vi "Yokogawa GX20 Acquire Continuous Measurement Data Example Ether Multiple.vi"() -> ()   [LabVIEW 2020]
doc: "This example shows how to configure multiple channels and acquire measurement data from multiple channels."
uses:
  <instrlib>/Yokogawa GX Series/Public/Data/Read Measurement Data (Analog NChan).vi
  <instrlib>/Yokogawa GX Series/Yokogawa GX Series.lvlib
panel:
  out "Chart":dbl[][](graph)
  in  "Parameters":T1(array[cluster])
  in  "Interval (1000)":u32=1000 min=25
  in  "Stop":bool
  # "(c) 2013-2018 Yokogawa Electric Corporation.  ALL RIGHTS RESERVED."
  # "ms"
  # "To execute this example, do below.\n1) Attach AI module to GX/GP/GM.\n2) Do Reconfiguring the GX/GP/GM (See User's Manual 1.24.2)\n3) Run this VI with valid VISA resource name (ex: \"TCPIP::192.168.0.2::34434::SOCKET\")"
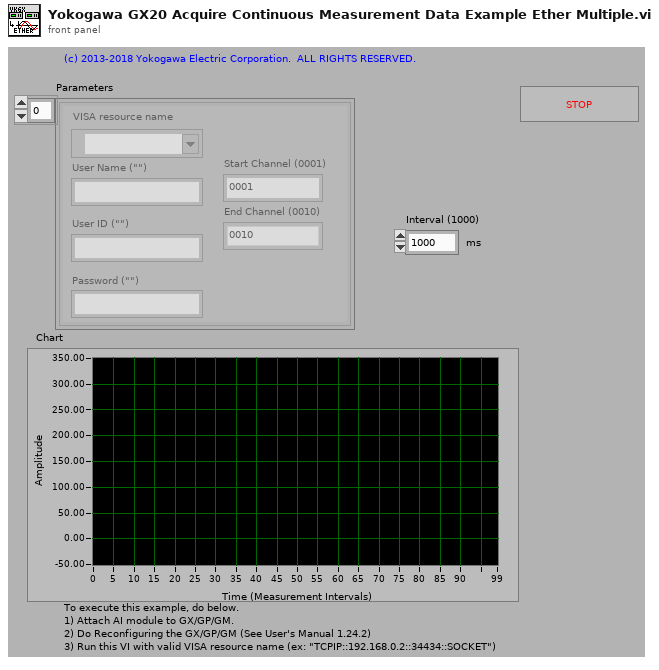
[diagram p1: front panel]
types:
  T1 = cluster{"VISA resource name":refnum<visa-resource-name>, "User Name (\"\")":string, "Password (\"\")":string, "Start Channel (0001) ":string, "End Channel (0010)":string, "User ID (\"\")":string}[]
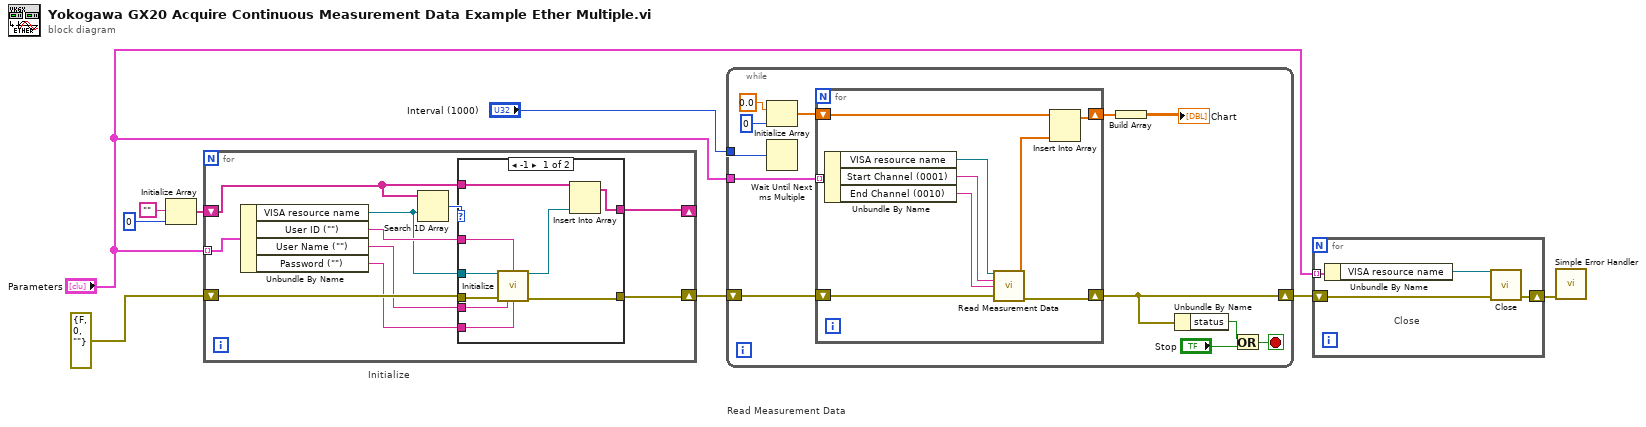
[diagram p0: block diagram]
diagram:
  # "Read Measurement Data"
  # "Initialize"
  n1 = Initialize Array("", 0) -> (w2:string[])
  n2 = for {
    tunnel: "Parameters" -> [w19] mode=indexing
    shift-right: [w17] -> w6
    shift-left: errorcluster {"status"=FALSE, "code"=0, "source"=""} ("error in (no error)") -> [w18]
    shift-right: [w14] -> _
    shift-left: w2 -> [w15]
    n3 = Unbundle By Name(w19) -> ("VISA resource name"=w10:refnum<visa-resource-name>, "User ID (\"\")"=w11:string, "User Name (\"\")"=w12:string, "Password (\"\")"=w13:string)
    n4 = Search 1D Array(1D array=w15, element=w10) -> (index of element=w16:i32)  [unwired: 1 in]
    n5 = case shown="-1" w16 {
      tunnel: w18 -> [w28 w29]
      tunnel: [w21 w29] -> w17
      tunnel: w12 -> [w27 _]
      tunnel: w13 -> [w26 _]
      tunnel: w10 -> [w25 _]
      tunnel: w15 -> [w24 w30]
      tunnel: [w23 w30] -> w14
      tunnel: w11 -> [w20 _]
      frame -1 {
        n6 = call <instrlib>:"Initialize.vi"("VISA resource name IN"=w25, "User ID (\"\")"=w20, "error in (no error)"=w28, "User Name (\"admin\")"=w27, "Password (\"\")"=w26) -> ("VISA resource name out"=w22:refnum<visa-resource-name>, "error out"=w21:errorcluster)  [unwired: 9 in]
        n7 = Insert Into Array(array=w24, new element=w22) -> (w23:string[])  [unwired: 1 in]
      }
      frame 0, Default {
      }
    }
  }
  n8 = while {
    shift-left: w6 -> [w38]
    shift-right: [w37] -> w9
    tunnel: "Interval (1000)" -> [w36]
    tunnel: "Parameters" -> [w39]
    stop <- w41 stop-if-true
    n9 = Initialize Array(0.0, 0) -> (w35:dbl[])
    n10 = Wait Until Next ms Multiple(millisecond multiple=w36) -> ()  [unwired: 1 out]
    n11 = for {
      tunnel: w39 -> [w51] mode=indexing
      shift-right: [w47] -> w37
      shift-left: w38 -> [w46]
      shift-right: [w43] -> w32
      shift-left: w35 -> [w45]
      n12 = Unbundle By Name(w51) -> ("VISA resource name"=w50:refnum<visa-resource-name>, "Start Channel (0001)"=w49:string, "End Channel (0010)"=w48:string)
      n13 = call-poly <instrlib>:"Read Measurement Data.vi"("VISA resource name"=w50, "Start Channel (1)"=w49, "End Channel (1)"=w48, "error in (no error)"=w46) -> ("Data"=w44:dbl[], "error out"=w47:errorcluster)  [unwired: 1 in, 9 out]
      n14 = Insert Into Array(array=w45, new element=w44) -> (w43:dbl[])  [unwired: 1 in]
    }
    n15 = Build Array(w32) -> (→"Chart":dbl[][])
    n16 = Unbundle By Name(w37) -> ("status"=w40:bool)
    n17 = Or(x=w40, y="Stop") -> (x .or. y?=w41:bool)
  }
  n18 = for {
    shift-right: [w53] -> w8
    shift-left: w9 -> [w54]
    tunnel: "Parameters" -> [w55] mode=indexing
    # "Close"
    n19 = Unbundle By Name(w55) -> ("VISA resource name"=w52:refnum<visa-resource-name>)
    n20 = call <instrlib>:"Close.vi"("error in (no error)"=w54, "VISA resource name"=w52) -> ("error out"=w53:errorcluster)  [unwired: 9 out]
  }
  n21 = call <vilib>:"Simple Error Handler.vi"("error in (no error)"=w8) -> ()  [unwired: 1 in, 8 out]
